vi "Displacement Table Number 2 Dataset Id.vi"(4 "Table Number":i32, 5 "Number of\nLBCBs":T3) -> (0 "Dataset Source":T1, 1 "Dataset Type":T2)   [LabVIEW 2009]
uses:
  Data Access Objects/Application/Number Of LBCBs.ctl
  Global Data/Transactions/Dataset Type.ctl
  Global Data/Transactions/Dataset Source.ctl
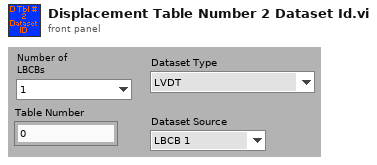
[diagram p1: front panel]
types:
  T1 = typedef "Dataset Source.ctl" = enum16{"LBCB 1", "LBCB 2", "Combined", "External Sensors"}
  T2 = typedef "Dataset Type.ctl" = enum16{"LVDT", "Load Cell", "Actuator Command", "Servo Error", "Displacement Command", "Displacement", "Force"}
  T3 = typedef "Number Of LBCBs.ctl" = enum16{"1", "2"}
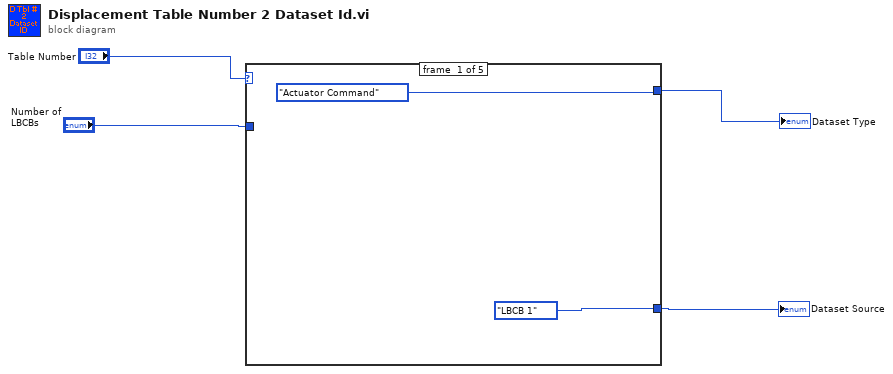
[diagram p0: block diagram]
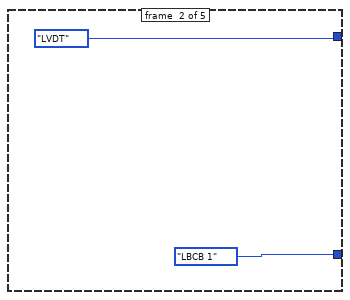
[diagram p2: hidden frame]
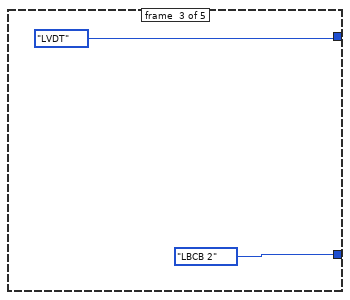
[diagram p3: hidden frame]
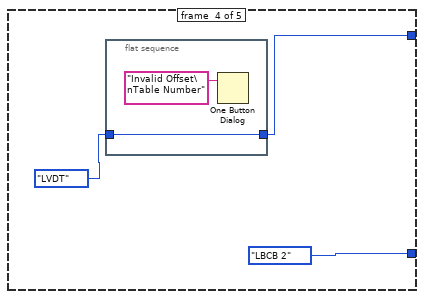
[diagram p4: hidden frame]
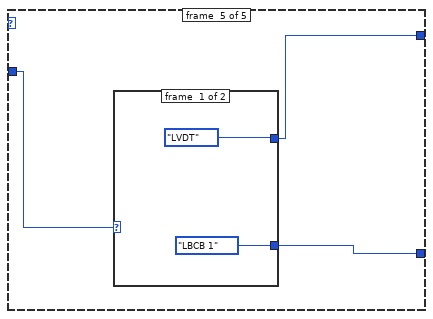
[diagram p5: hidden frame]
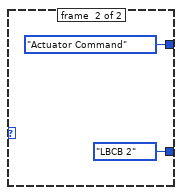
[diagram p6: hidden frame]
diagram:
  n1 = case shown="1" "Table Number" {
    tunnel: [Dataset_Source."LBCB 1" ("Dataset Source") Dataset_Source."LBCB 1" ("Dataset Source") Dataset_Source."LBCB 2" ("Dataset Source") Dataset_Source."LBCB 2" ("Dataset Source") w18] -> w2
    tunnel: [Dataset_Type."Actuator Command" ("Dataset Type") Dataset_Type."LVDT" ("Dataset Type") Dataset_Type."LVDT" ("Dataset Type") w11 w16] -> w3
    tunnel: "Number of\nLBCBs" -> [_ _ _ _ w17]
    frame #0 {
    }
    frame #1 {
    }
    frame #2 {
    }
    frame #3 {
      n2 = flat-sequence {
        tunnel: Dataset_Type."LVDT" ("Dataset Type") -> [w15]
        tunnel: [w15] -> w11
        frame #0 {
          n3 = One Button Dialog(message="Invalid Offset\nTable Number") -> ()  [unwired: 1 in, 1 out]
        }
      }
    }
    frame #4 {
      n4 = case shown="\"2\"" w17 {
        tunnel: [Dataset_Source."LBCB 1" ("Dataset Source") Dataset_Source."LBCB 2" ("Dataset Source")] -> w18
        tunnel: [Dataset_Type."LVDT" ("Dataset Type") Dataset_Type."Actuator Command" ("Dataset Type")] -> w16
        frame #0 {
        }
        frame #1 {
        }
      }
    }
  }
  "Dataset Type" <- w3
  "Dataset Source" <- w2
